vi "Averaged_Rot_Measure_Main_v3_gradient_comp.vi"() -> ()   [LabVIEW 2021]
uses:
  Config_File_Paths.ctl
  ZI_Data.ctl
  <vilib>/Analysis/baseanly.llb/Mean (DBL).vi
  <vilib>/measure/maspectr.llb/FFT Spectrum (Real-Im) for 1 Chan.vi
  <vilib>/Analysis/NI_AALPro.lvlib
  <vilib>/measure/NI_MAPro.lvlib
  <vilib>/Analysis/NI_AALBase.lvlib
panel:
  out "single differ 3":cluster{"Time":dbl[], "X":dbl[]}[](graph)
  out "output array":dbl[][](array[numeric])
  out "Waveform Graph 2":waveform(dbl)(graph)
  out "Array":dbl[](array[numeric])
  out "Waveform Graph":waveform(dbl)[](graph)
  out "Possible Mismatch In Phase (?)":bool
  out "Enough Points (?)":bool
  out "Trig Out Found(?)":bool
  out "Meter":dbl(knob) scale=-15.0..15.0
  out "single abs\nspectrum":waveform(dbl)(graph)
  out "single rot \nspectrum":waveform(dbl)[](graph)
  out "single differ":cluster{"Time":dbl[], "X":dbl[]}[](graph)
  out "single abs":cluster{"Time":dbl[], dbl[]}(graph)
  out "single rot":cluster{"Time":dbl[], "X":dbl[]}[](graph)
  in  "Resource Address":T1={"ZI Address"="DEV714", "VISA Keithley"="KEITHLEY", "VISA Arduino PG"="ARDUINO"}
  in  "error in":errorcluster
  in  "Config files paths":T2={"ZI config file (.ini)"="Config_Ver_1\\Zurich_params.ini", "Keithley config file (.ini)"="Config_Ver_1\\Keithley_params.ini", "Arduino config file (.ini)"="Config_Ver_1\\pulse_sequence.ini"}
  in  "Time unit":string(combo)="us"
  out "loading":dbl(slide) scale=0.0..100.0
  in  "Number of averages":i32=1
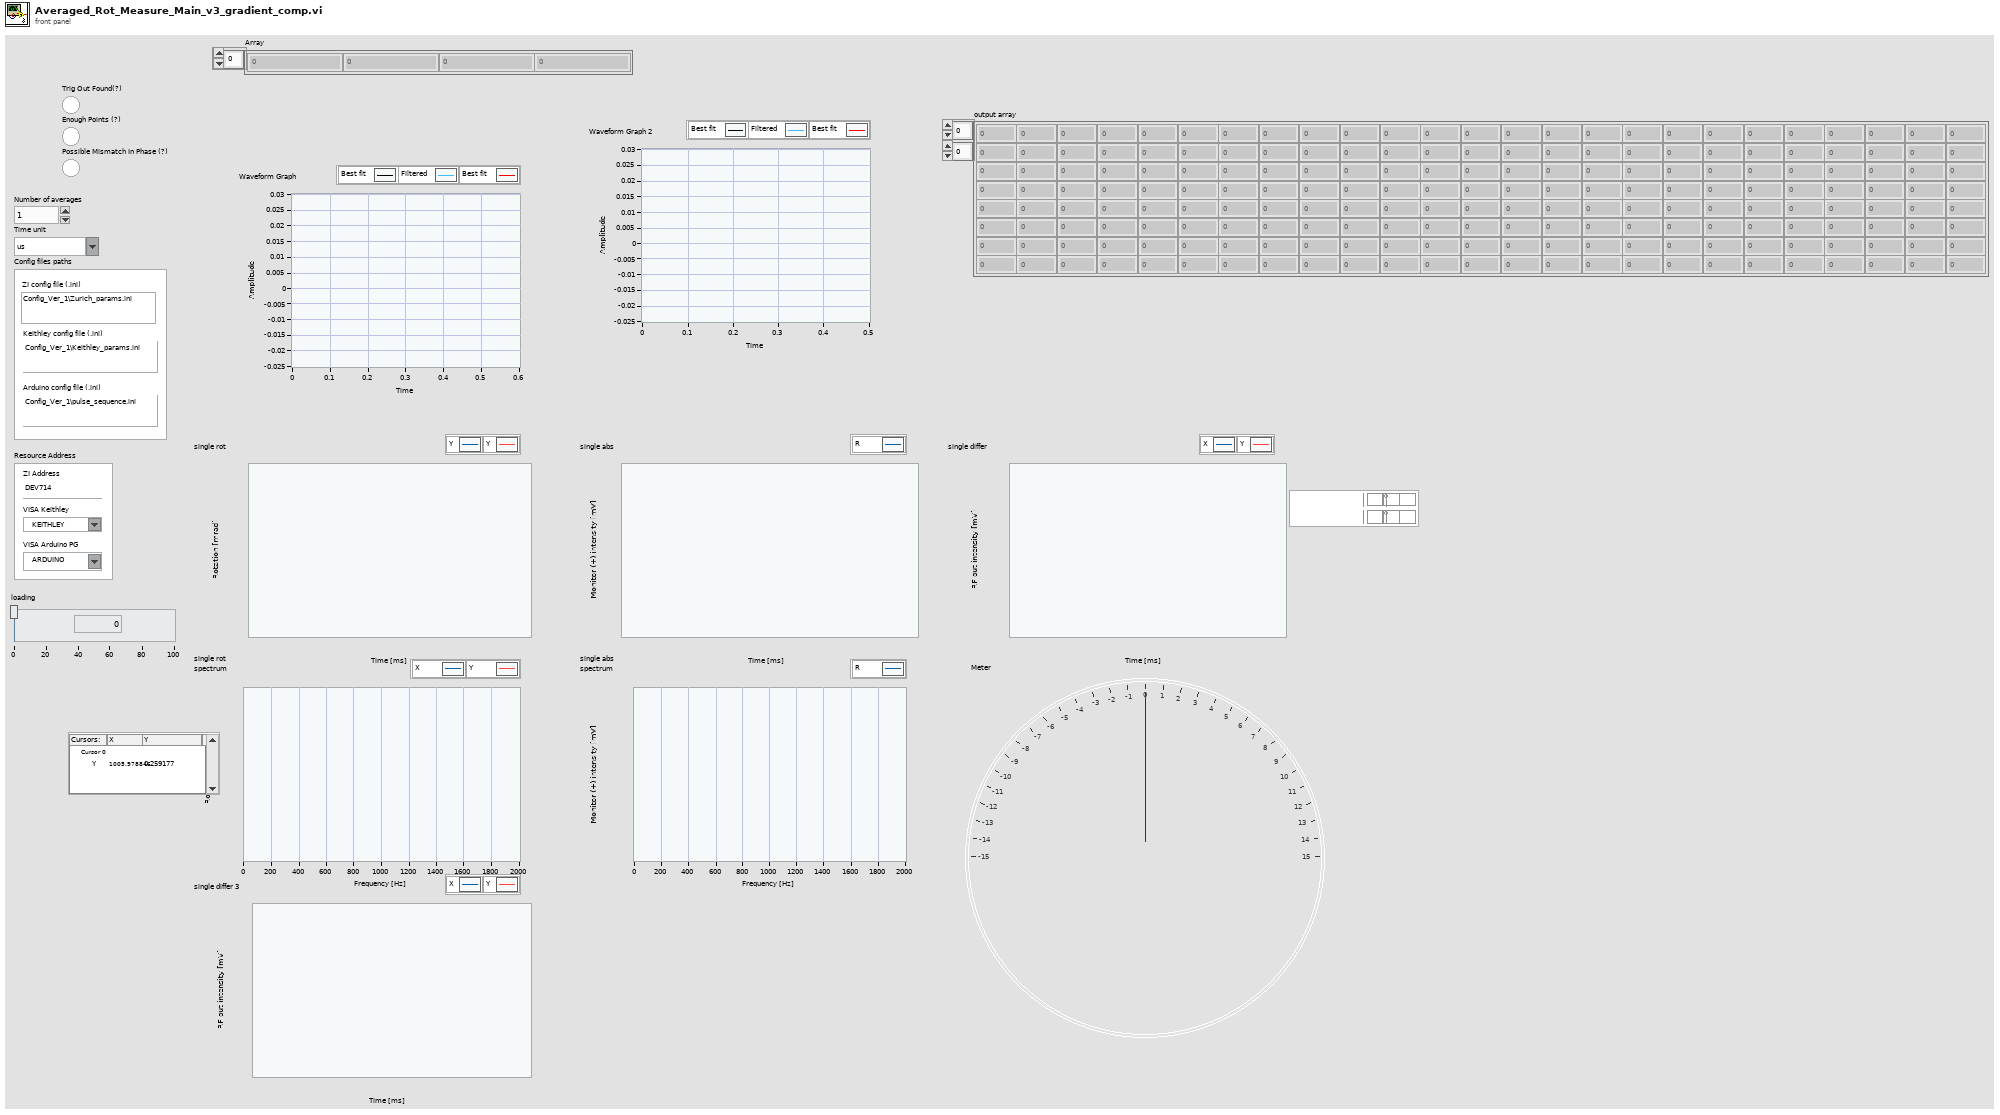
[diagram p1: front panel]
types:
  T1 = cluster{"ZI Address":string, "VISA Keithley":refnum<visa-resource-name>, "VISA Arduino PG":refnum<visa-resource-name>}
  T2 = typedef "Config_File_Paths.ctl" = cluster{"ZI config file (.ini)":string, "Keithley config file (.ini)":string, "Arduino config file (.ini)":string}
  T3 = typedef "ZI_Data.ctl" = cluster{"R":dbl[], "Theta":dbl[], "X":dbl[], "Y":dbl[], "AuxIn0":dbl[], "AuxIn1":dbl[], "Frequency":dbl[], "DIO":dbl[], "Time":dbl[]}
  T4 = typedef "Resources.ctl" = cluster{"ZI Handle":T5, "ZI ModHandle":T6, "VISA arduino":refnum<visa-resource-name>, "VISA Keithley":refnum<visa-resource-name>}
  T5 = typedef "Zurich Instruments LabOne.lvlib/ziTypeHandle.ctl" = cluster{"handleValid":bool, "Conn":u64, "Path Prefix":string, "Handle":u64, "Connected":bool, "Clockbase(s)":dbl}
  T6 = typedef "Zurich Instruments LabOne.lvlib/ziTypeModHandle.ctl" = cluster{"handleValid":bool, "Conn":u64, "ModHandle":u64, "moduleID":string, "Path Prefix":string}
  T7 = typedef "Cutted_Data.ctl" = cluster{"X":dbl[], "Y":dbl[], "Time":dbl[]}
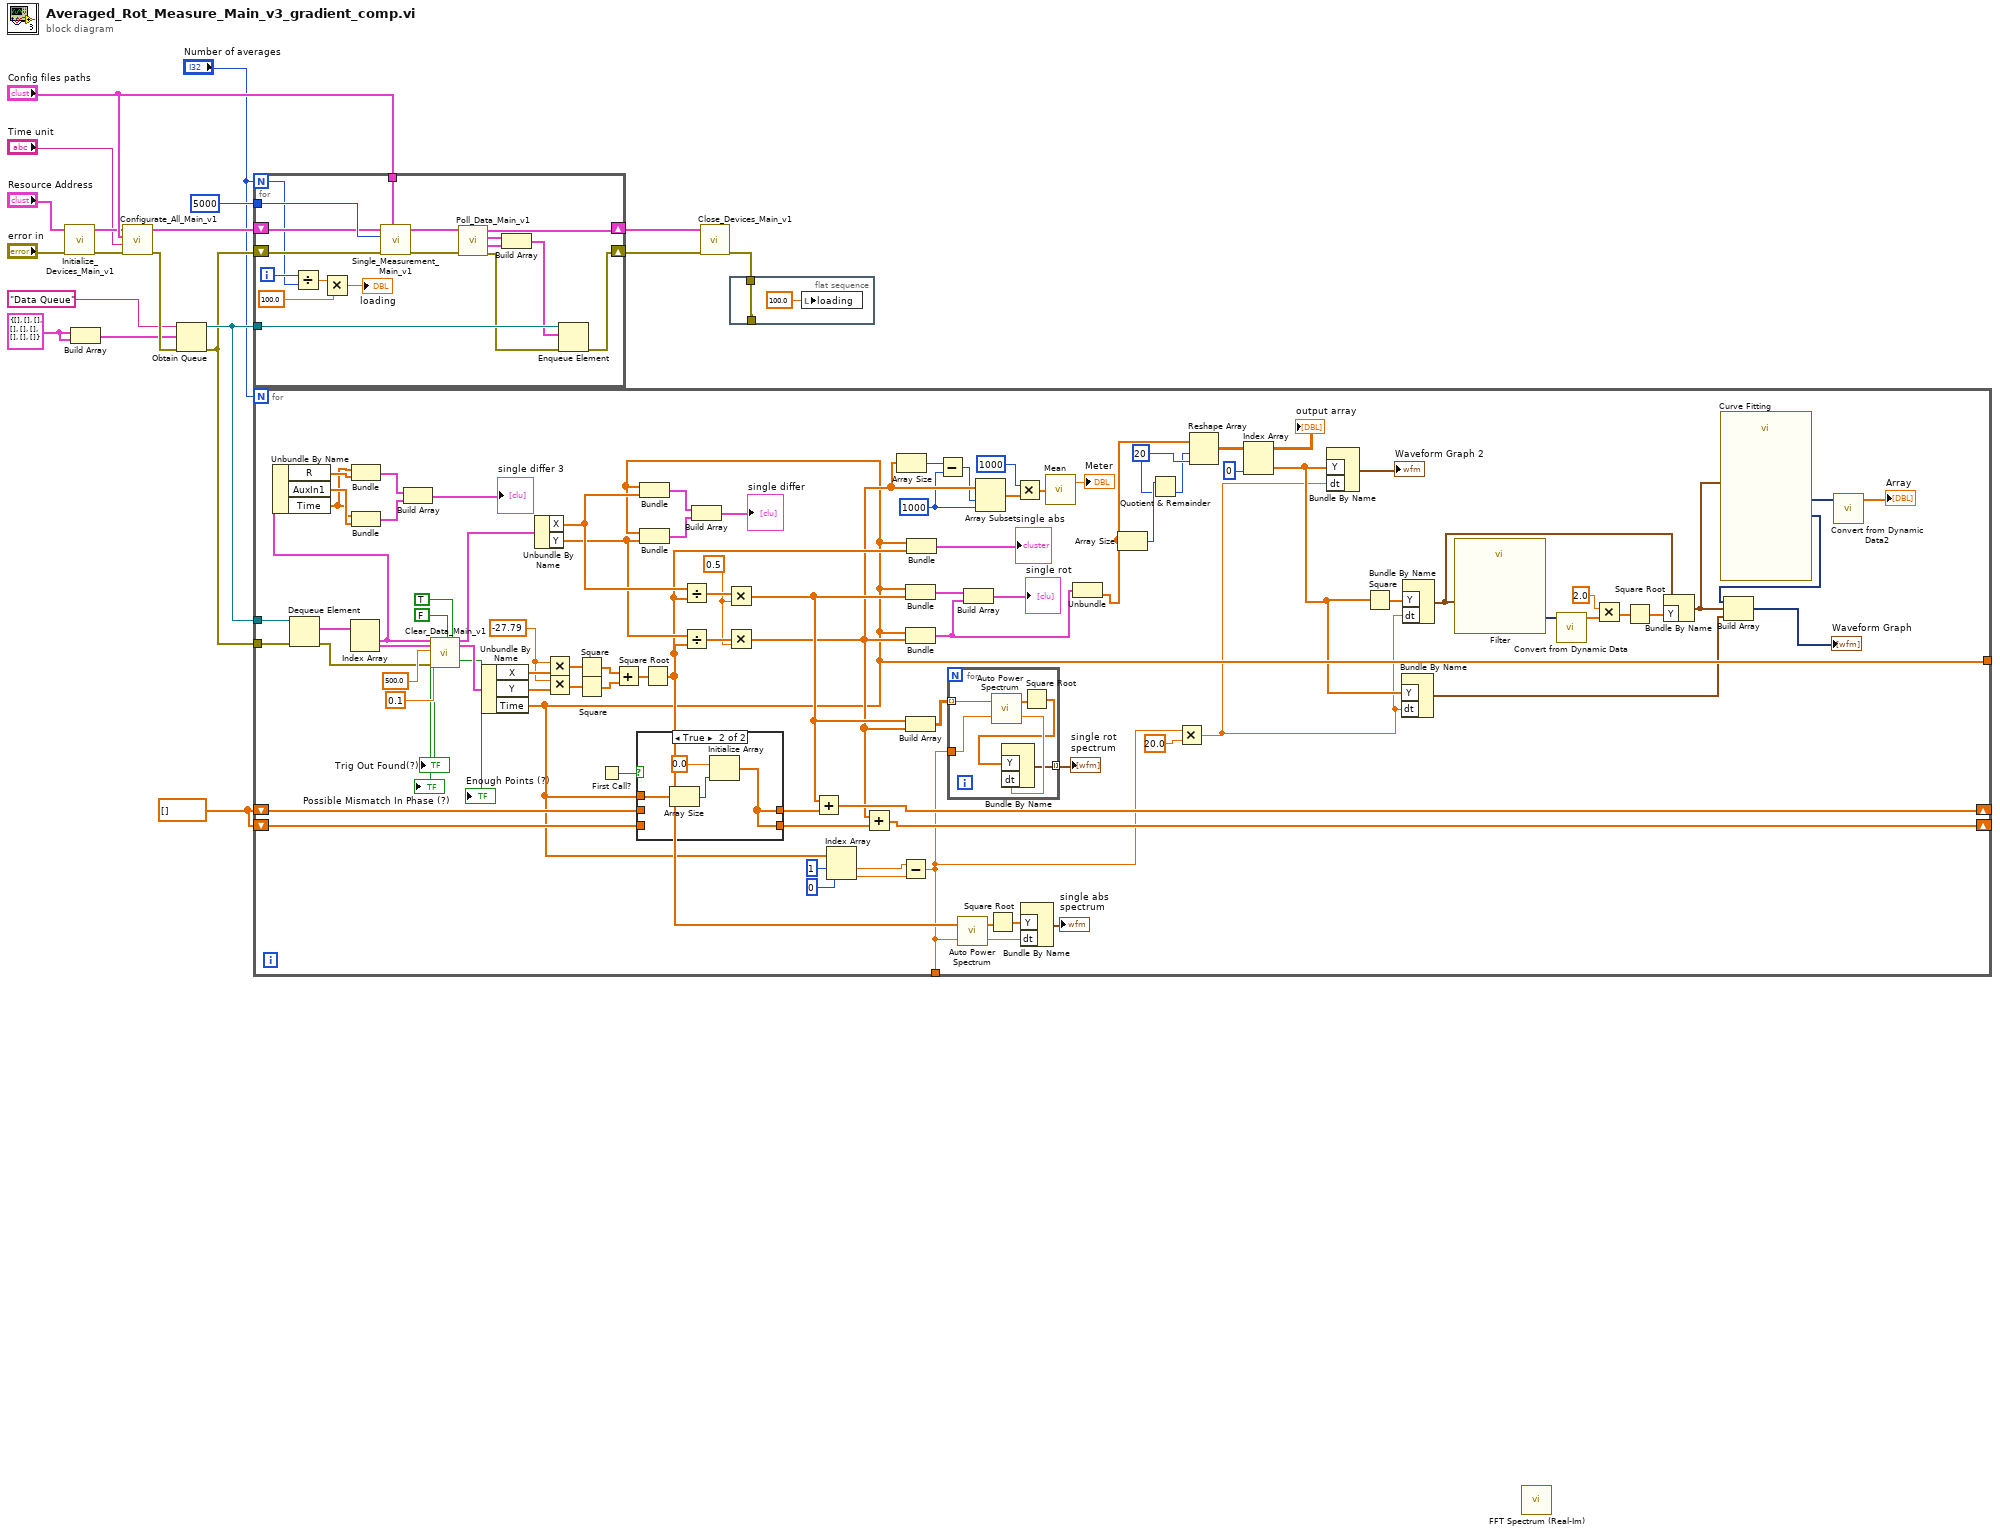
[diagram p0: block diagram]
diagram:
  w3 = dbl[] []
  w7 = T3 {"R"=[], "Theta"=[], "X"=[], "Y"=[], "AuxIn0"=[], "AuxIn1"=[], "Frequency"=[], "DIO"=[], "Time"=[]} ("ZI Data")
  n1 = call "Initialize_Devices_Main_v1.vi"("error in"="error in", "Resource Address"="Resource Address") -> ("error out"=w11:errorcluster, "Resources"=w12:T4)  [unwired: 8 in]
  n2 = Build Array(w7, w7) -> (w6:T3[])
  n3 = call "Configurate_All_Main_v1.vi"("error in"=w11, "Time unit"="Time unit", "Config files paths"="Config files paths", "Resources in"=w12) -> ("error out"=w9:errorcluster, "Resources out"=w17:T4)  [unwired: 4 in, 2 out]
  n4 = Obtain Queue(name (unnamed)="Data Queue", element data type=w6, error in (no error)=w9) -> (queue out=w5:refnum<queue>, error out=w4:errorcluster)  [unwired: 2 in, 1 out]
  n5 = for {
    N: "Number of averages" -> [w29]
    shift-right: [w31] -> w18
    shift-left: w17 -> [w35]
    shift-right: [w20] -> w19
    shift-left: w4 -> [w34]
    tunnel: "Config files paths" -> [w37]
    tunnel: u64 5000 ("Timeout [ms]") -> [w36]
    tunnel: w5 -> [w25]
    i -> [w30]
    n6 = Divide(x=w30, y=w29) -> (x/y=w28:dbl)
    n7 = Multiply(x=w28, y=100.0) -> (x*y=→"loading":dbl)
    n8 = call "Single_Measurement_Main_v1.vi"("Config files paths"=w37, "error in"=w34, "Timeout [ms]"=w36, "Resources In"=w35) -> ("error out"=w32:errorcluster, "Resources Out"=w33:T4)  [unwired: 6 in]
    n9 = call "Poll_Data_Main_v1.vi"("error in"=w32, "Resources in"=w33) -> ("error out"=w21:errorcluster, "ZI Data 3"=w23:T3, "ZI Data 0"=w24:T3, "Resources out"=w31:T4)  [unwired: 6 in]
    n10 = Build Array(w24, w23) -> (w22:T3[])
    n11 = Enqueue Element(queue=w25, element=w22, error in (no error)=w21) -> (error out=w20:errorcluster)  [unwired: 1 in, 2 out]
  }
  n12 = for {
    N: "Number of averages" -> [_]
    tunnel: w5 -> [w130]
    tunnel: w4 -> [w129]
    shift-right: [w114] -> _
    shift-left: w3 -> [w118]
    shift-right: [w113] -> _
    shift-left: w3 -> [w117]
    tunnel: [w65] -> _
    tunnel: [w48] -> _
    w42 = 20 ("dimension size")
    w80 = 1000 ("length")
    w102 = 0.5
    w105 = -27.79
    n13 = Dequeue Element(queue=w130, error in (no error)=w129) -> (element=w128:T3[], error out=w124:errorcluster)  [unwired: 1 in, 2 out]
    n14 = Index Array(array=w128) -> (element #1=w71:T3, element #2=w127:T3)  [unwired: 2 in]
    n15 = Unbundle By Name(w71) -> ("R"=w68:dbl[], "AuxIn1"=w67:dbl[], "Time"=w66:dbl[])
    n16 = Bundle("Time"=w66, "R"=w68) -> (w70:cluster{"Time":dbl[], "R":dbl[]})  [unwired: 1 in]
    n17 = Bundle("Time"=w66, "AuxIn1"=w67) -> (w69:cluster{"Time":dbl[], "AuxIn1":dbl[]})  [unwired: 1 in]
    n18 = Build Array(w70, w69) -> (→"single differ 3":cluster{"Time":dbl[], "AuxIn1":dbl[]}[])
    n19 = call "Clear_Data_Main_v1.vi"("ZI Data 0"=w71, "ZI Data 3"=w127, "Time Of Collected Data (ms)"=500.0, "Crosstalk Tolerance"=0.1, "error in"=w124, "Fixed Number Of Points"=FALSE, "Check Phase Mismatch"=TRUE) -> ("Trig Out Found(?)"=→"Trig Out Found(?)":bool, "Enough Points (?)"=→"Enough Points (?)":bool, "Possible Mismatch In Phase (?)"=→"Possible Mismatch In Phase (?)":bool, "Cutted Data"=w121:T7, "Cutted Data 3"=w120:T7)  [unwired: 7 in, 1 out]
    n20 = Unbundle By Name(w120) -> ("X"=w106:dbl[], "Y"=w107:dbl[], "Time"=w65:dbl[])
    n21 = Unbundle By Name(w121) -> ("X"=w108:dbl[], "Y"=w95:dbl[])
    n22 = Multiply(x=w105, y=w106) -> (x*y=w91:dbl[])
    n23 = Multiply(x=w105, y=w107) -> (x*y=w90:dbl[])
    n24 = Square(x=w91) -> (x^2=w93:dbl[])
    n25 = Square(x=w90) -> (x^2=w92:dbl[])
    n26 = First Call?() -> (First Call?: T/F=w119:bool)
    n27 = Add(x=w93, y=w92) -> (x+y=w94:dbl[])
    n28 = case shown="True" w119 {
      tunnel: w65 -> [_ w142]
      tunnel: w118 -> [w138 _]
      tunnel: [w138 w139] -> w115
      tunnel: [w137 w139] -> w116
      tunnel: w117 -> [w137 _]
      frame False {
      }
      frame True {
        n29 = Array Size(array=w142) -> (size(s)=w140:i32)
        n30 = Initialize Array(0.0 ("element"), w140) -> (w139:dbl[])
      }
    }
    n31 = Bundle("Time"=w65, "X"=w108) -> (w111:cluster{"Time":dbl[], "X":dbl[]})  [unwired: 1 in]
    n32 = Bundle("Time"=w65, "Y"=w95) -> (w110:cluster{"Time":dbl[], "Y":dbl[]})  [unwired: 1 in]
    n33 = Square Root(x=w94) -> (sqrt(x)=w85:dbl[])
    n34 = Divide(x=w108, y=w85) -> (x/y=w104:dbl[])
    n35 = Divide(x=w95, y=w85) -> (x/y=w103:dbl[])
    n36 = Build Array(w111, w110) -> (→"single differ":cluster{"Time":dbl[], "Y":dbl[]}[])
    n37 = Multiply(x=w104, y=w102) -> (x*y=w88:dbl[])
    n38 = Multiply(x=w103, y=w102) -> (x*y=w81:dbl[])
    n39 = Add(x=w88, y=w115) -> (x+y=w114:dbl[])
    n40 = Index Array(array=w65, index #1=1 ("index"), index #2=0 ("index")) -> (element #1=w98:dbl, element #2=w97:dbl)
    n41 = Add(x=w81, y=w116) -> (x+y=w113:dbl[])
    n42 = Array Size(array=w81) -> (size(s)=w79:i32)
    n43 = Subtract(x=w98, y=w97) -> (x-y=w48:dbl)
    n44 = Bundle("Time"=w65, w88) -> (w64:cluster{"Time":dbl[], dbl[]})  [unwired: 1 in]
    n45 = Bundle("Time"=w65, w81) -> (w63:cluster{"Time":dbl[], dbl[]})  [unwired: 1 in]
    n46 = Build Array(w88, w81) -> (w101:dbl[][])
    n47 = Bundle("Time"=w65, w85) -> (→"single abs":cluster{"Time":dbl[], dbl[]})  [unwired: 1 in]
    n48 = Subtract(x=w79, y=w80) -> (x-y=w78:i32)
    n49 = for {
      tunnel: w101 -> [w136] mode=indexing
      tunnel: w48 -> [w135]
      tunnel: [w133] -> w96 mode=indexing
      n50 = call <vilib>:"Auto Power Spectrum.vi"("dt"=w135, "Signal (V)"=w136) -> ("df"=w134:dbl, "Power Spectrum (V^2 rms)"=w132:dbl[])
      n51 = Square Root(x=w132) -> (sqrt(x)=w131:dbl[])
      n52 = Bundle By Name("Y"=w131, "dt"=w134) -> (w133:waveform(dbl))  [unwired: 1 in]
    }
    "single rot \nspectrum" <- w96
    n53 = call <vilib>:"Auto Power Spectrum.vi"("dt"=w48, "Signal (V)"=w85) -> ("df"=w86:dbl, "Power Spectrum (V^2 rms)"=w87:dbl[])
    n54 = Build Array(w64, w63) -> (→"single rot":cluster{"Time":dbl[], dbl[]}[])
    n55 = Array Subset(array=w81, index=w78, length=w80) -> (w77:dbl[])
    n56 = Square Root(x=w87) -> (sqrt(x)=w84:dbl[])
    n57 = Multiply(x=1000, y=w77) -> (x*y=w75:dbl[])
    n58 = Bundle By Name("Y"=w84, "dt"=w86) -> (→"single abs\nspectrum":waveform(dbl))  [unwired: 1 in]
    n59 = call-poly <vilib>:"Mean.vi"("X"=w75) -> ("mean"=→"Meter":dbl)  [unwired: 1 out]
    n60 = Unbundle(w63) -> (w49:dbl[])  [unwired: 1 out]
    n61 = Array Size(array=w49) -> (size(s)=w45:i32)
    n62 = Quotient & Remainder(x=w45, y=w42) -> (floor(x/y)=w41:i32)  [unwired: 1 out]
    n63 = Multiply(x=w48, y=20.0) -> (x*y=w39:dbl)
    n64 = Reshape Array(w49, w41, w42) -> (w47:dbl[][])
    "output array" <- w47
    n65 = Index Array(array=w47, index (col)=0 ("disabled index (col)")) -> (element=w40:dbl[])  [unwired: 1 in]
    n66 = Bundle By Name("Y"=w40, "dt"=w39) -> (→"Waveform Graph 2":waveform(dbl))  [unwired: 1 in]
    n67 = Square(x=w40) -> (x^2=w50:dbl[])
    n68 = Bundle By Name("Y"=w40, "dt"=w39) -> (w46:waveform(dbl))  [unwired: 1 in]
    n69 = Bundle By Name("Y"=w50, "dt"=w39) -> (w58:waveform(dbl))  [unwired: 1 in]
    n70 = call "Filter"("Signal"=w58) -> ("Filtered Signal"=w61:dynamicdata)  [unwired: 9 in, 1 out]
    n71 = call "Convert from Dynamic Data"("Dynamic Data Type"=w61) -> ("Array"=w60:dbl[])  [unwired: 3 in]
    n72 = Multiply(x=2.0, y=w60) -> (x*y=w57:dbl[])
    n73 = Square Root(x=w57) -> (sqrt(x)=w56:dbl[])
    n74 = Bundle By Name(cluster=w58, "Y"=w56) -> (w54:waveform(dbl))
    n75 = call "Curve Fitting"("Signals"=w54) -> ("best fit"=w55:dynamicdata, "non-linear coefficients"=w53:dynamicdata)  [unwired: 6 in, 3 out]
    n76 = Build Array(w55, w54, w46) -> (→"Waveform Graph":dynamicdata[])
    n77 = call "Convert from Dynamic Data2"("Dynamic Data Type"=w53) -> ("Array"=→"Array":dbl[])  [unwired: 3 in]
  }
  n78 = call "Close_Devices_Main_v1.vi"("error in"=w19, "Resources in"=w18) -> ("error out"=w1:errorcluster)  [unwired: 9 in]
  n79 = flat-sequence {
    tunnel: [w143] -> _
    tunnel: w1 -> [w143]
    frame #0 {
      n80 = local write "loading"(100.0 ("loading")) -> ()
    }
  }
  n81 = call-poly <vilib>:"FFT Spectrum (Real-Im).vi"() -> ()  [unwired: 7 in, 5 out]
